vi "Version 1_Write SetPoint.vi"(6 "Software Version (Optional - wire for speed)":u8, 7 "Address (A)":string="A", 8 "error in":errorcluster, 9 "Setpoint":dbl format="%_4g", 10 "Controller Info in":T1={"Controller Select"=enum."Unknown", "fullscale"=nan, "Control Range"=enum."Unknown"} {"fullscale" format="%_4g"}, 11 "VISA Session In":refnum<visa-resource-name>="Alicat") -> (0 "error out":errorcluster, 2 "Controller Info out (Not all controller select\nvariables can be shown in version 1's output)":T1={"Controller Select"=enum."Unknown", "fullscale"=nan, "Control Range"=enum."Unknown"} {"fullscale" format="%_4g"}, 3 "VISA Session Out":refnum<visa-resource-name>)   [LabVIEW 2015]
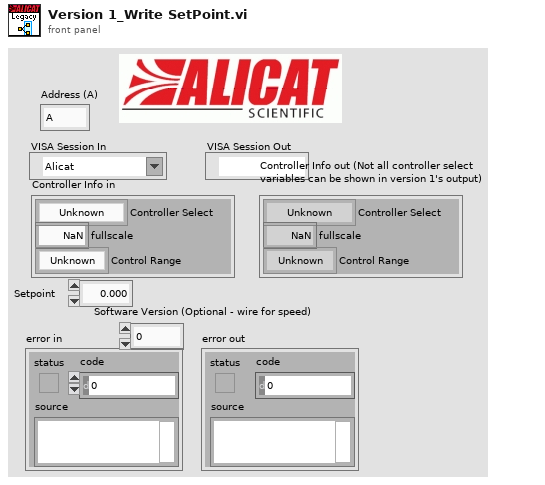
[diagram p1: front panel]
types:
  T1 = cluster{"Controller Select":enum8{"No controller", "Pressure", "Temperature", "Volumetric Flow", "Mass Flow", "Unknown"}, "fullscale":dbl, "Control Range":enum16{"Normal", "Invert", "Bipolar", "Unknown"}}
  T2 = enum8{"No controller", "Pressure", "Temperature", "Volumetric Flow", "Mass Flow", "Unknown"}
  T3 = cluster{"Controller Full Scale":dbl, "Controller Select":u16, "Control Range":enum16{"Normal", "Inverted", "Bidirectional", "Unknown"}}
  T4 = enum16{"Normal", "Inverted", "Bidirectional", "Unknown"}
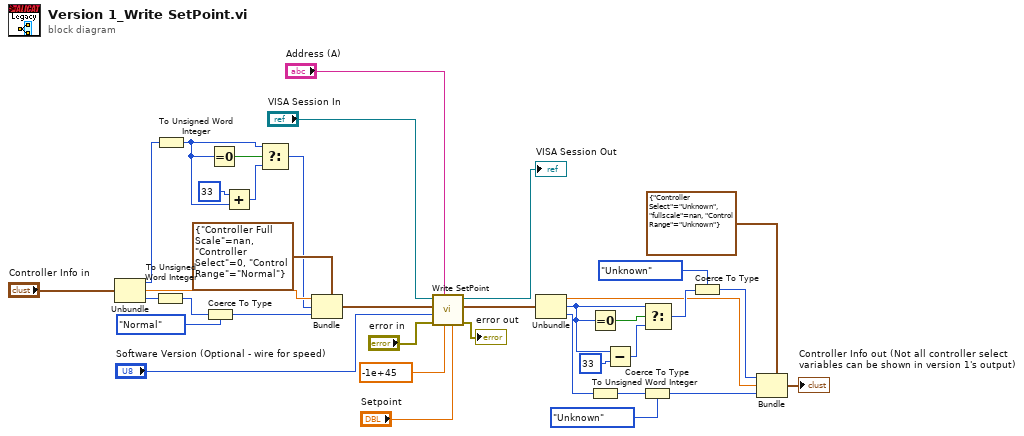
[diagram p0: block diagram]
diagram:
  n1 = Unbundle("Controller Info in") -> ("Controller Select"=w19:T2, "fullscale"=w29:dbl, "Control Range"=w28:enum16{"Normal", "Invert", "Bipolar", "Unknown"})
  n2 = To Unsigned Word Integer(number=w28) -> (unsigned 16bit integer=w26:u16)
  n3 = To Unsigned Word Integer(number=w19) -> (unsigned 16bit integer=w21:u16)
  n4 = Coerce To Type(0:w26, 1:T4."Normal" ("Control Range")) -> (2:w25:T4)
  n5 = Equal To 0?(x=w21) -> (x = 0?=w22:bool)
  n6 = Add(x=u16 33, y=w21) -> (x+y=w20:u16)
  n7 = Select(t=w21, s=w22, f=w20) -> (s? t:f=w18:u16)
  n8 = Bundle(cluster=T3 {"Controller Full Scale"=nan, "Controller Select"=0, "Control Range"=enum."Normal"} ("Controller Info out"), "Controller Full Scale"=w29, "Controller Select"=w18, "Control Range"=w25) -> (w17:T3)
  n9 = call "Write SetPoint.vi"("Setpoint"="Setpoint", "Previous Setpoint"=-1e+45, "Unit ID (A)"="Address (A)", "error in"="error in", "Software Version"="Software Version (Optional - wire for speed)", "Controller Info out"=w17, "VISA Session In"="VISA Session In") -> ("error out"=→"error out":errorcluster, "Controller Info out"=w16:T3, "VISA Session Out"=→"VISA Session Out":refnum<visa-resource-name>)  [unwired: 1 in, 1 out]
  n10 = Unbundle(w16) -> ("Controller Full Scale"=w5:dbl, "Controller Select"=w9:u16, "Control Range"=w4:T4)
  n11 = Equal To 0?(x=w9) -> (x = 0?=w11:bool)
  n12 = To Unsigned Word Integer(number=w4) -> (unsigned 16bit integer=w3:u16)
  n13 = Subtract(x=w9, y=u16 33 ("x")) -> (x-y=w10:u16)
  n14 = Coerce To Type(0:w3, 1:enum16{"Normal", "Invert", "Bipolar", "Unknown"}."Unknown" ("Control Range")) -> (2:w1:enum16{"Normal", "Invert", "Bipolar", "Unknown"})
  n15 = Select(t=w9, s=w11, f=w10) -> (s? t:f=w8:u16)
  n16 = Coerce To Type(0:w8, 1:T2."Unknown" ("Controller Select")) -> (2:w6:T2)
  n17 = Bundle(cluster=T1 {"Controller Select"=enum."Unknown", "fullscale"=nan, "Control Range"=enum."Unknown"} ("Controller Info out"), "Controller Select"=w6, "fullscale"=w5, "Control Range"=w1) -> (→"Controller Info out (Not all controller select\nvariables can be shown in version 1's output)":T1)
